vi "Write Mail To Next Actor.vi"(8 "error in (no error)":errorcluster, 10 "Mail Strategy.lvclass":refnum<class "Mail Strategy.lvclass">, 11 "Composite Task in":refnum<class "Composite Task.lvclass">) -> (0 "error out":errorcluster, 3 "Composite Task out":refnum<class "Composite Task.lvclass">)   [LabVIEW 2019, in "Composite Task.lvclass"]
uses:
  Composite Task.lvclass
  Messenger/Mail Strategy/Mail Strategy.lvclass
  Composite Task.lvclass/Composite Task.ctl
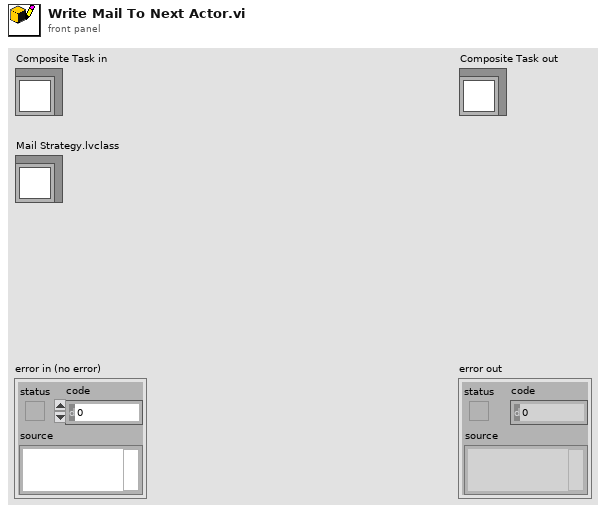
[diagram p1: front panel]
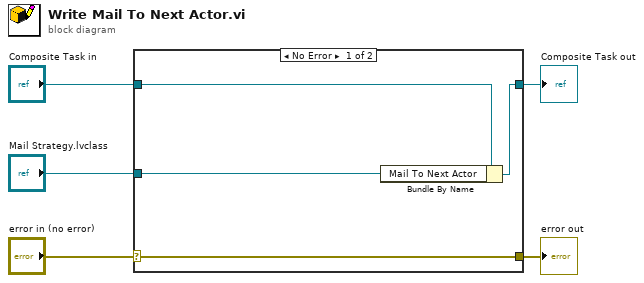
[diagram p0: block diagram]
diagram:
  n1 = case shown="No Error" "error in (no error)" {
    selector: "error in (no error)" -> [w9 w10]
    tunnel: [w9 w10] -> w4
    tunnel: [w7 w11] -> w2
    tunnel: "Composite Task in" -> [w8 w11]
    tunnel: "Mail Strategy.lvclass" -> [w6 _]
    frame No Error {
      n2 = Bundle By Name(cluster=w8, "Mail To Next Actor"=w6) -> (w7:refnum<class "Composite Task.lvclass">)
    }
    frame Error {
    }
  }
  "error out" <- w4
  "Composite Task out" <- w2
